vi "CLD 9 Step Sequencer Express Timer Solution.vi"() -> ()   [LabVIEW 2019]
doc: "CLD 9\n\nThis solution uses the Express VI Elapsed Time as a method for timing the changing of states. All of the stat data is hard coded for this exercise."
uses:
  CLD 9 Timer Enum.ctl
panel:
  out "Current Step Time":dbl
  out "Elapsed Time (s)":dbl format="%#.1g"
  out "Step 3":bool
  out "Step 2":bool
  out "Step 1":bool
  out "Time Has Elapsed":bool
  in  "Auto Reset":bool=TRUE
  in  "Reset Button":bool
  in  "Stop VI":bool
  out "error out":errorcluster
  in  "error in":errorcluster
  in  "Time Target (s)":dbl
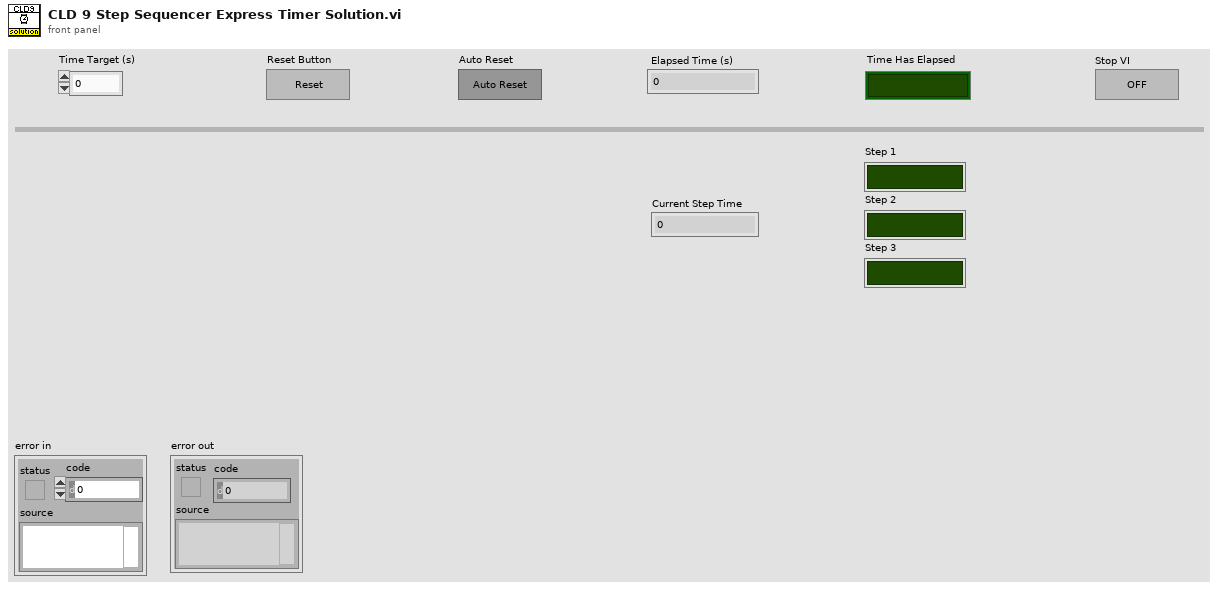
[diagram p1: front panel]
types:
  T1 = typedef "CLD 9 Timer Enum.ctl" = enum16{"Start Step One", "Run Step One", "Start Step Two", "Run Step Two", "Start Step Three", "Run Step Three"}
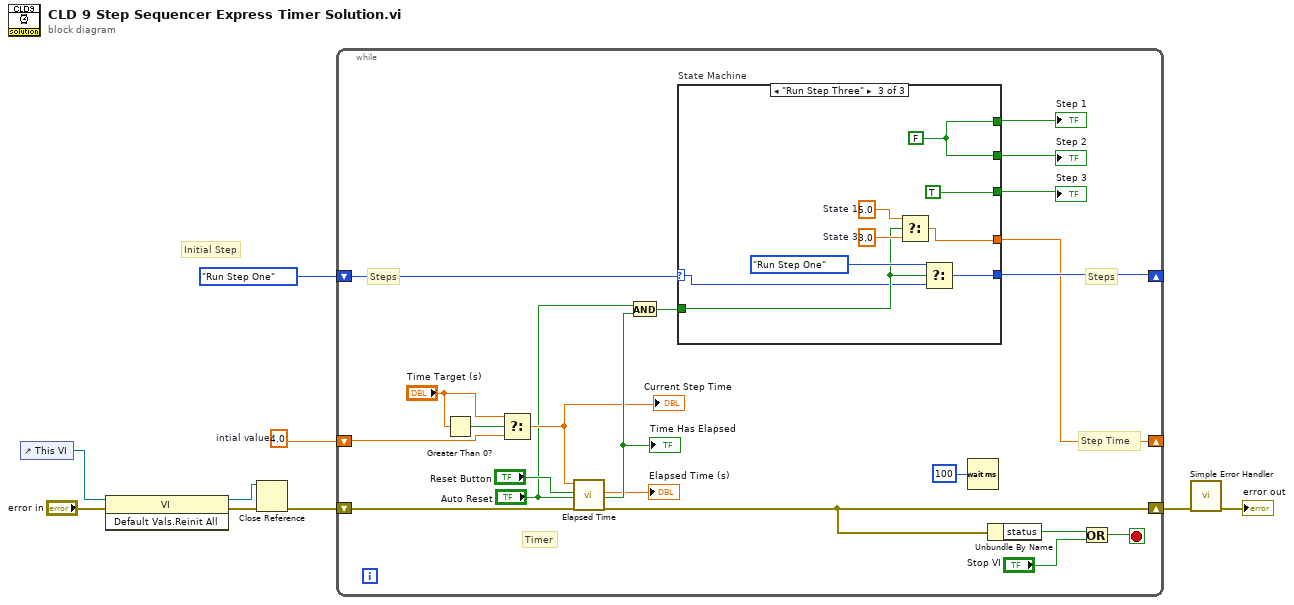
[diagram p0: block diagram]
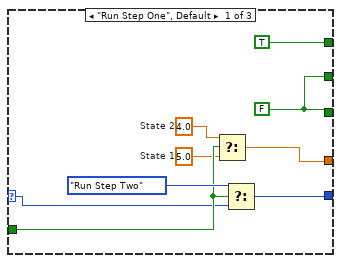
[diagram p2: hidden frame]
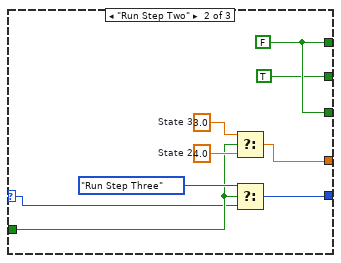
[diagram p3: hidden frame]
diagram:
  w1 = 4.0  # intial value
  # "Initial Step"
  n1 = control-ref of="This VI"() -> (w5:refnum<vi>)
  n2 = invoke class="VI" method="Default Vals.Reinit All"(reference=w5, error in="error in") -> (reference out=w3:refnum<vi>, error out=w6:errorcluster)  [unwired: 1 in, 1 out]
  n3 = Close Reference(reference=w3, error in (no error)=w6) -> (error out=w4:errorcluster)
  n4 = while {
    shift-right: [w13] -> w8
    shift-left: w4 -> [w28]
    shift-right: [w26] -> _
    shift-left: CLD_9_Timer_Enum."Run Step One" ("Enum") -> [w25]
    shift-right: [w17] -> _
    shift-left: w1 -> [w16]
    stop <- w12 stop-if-true
    # "Timer"
    # "Steps"
    # "Steps"
    # "Step Time"
    n5 = Greater Than 0?(x="Time Target (s)") -> (x > 0?=w20:bool)
    n6 = Select(t="Time Target (s)", s=w20, f=w16) -> (s? t:f=w18:dbl)
    "Current Step Time" <- w18
    n7 = call "Elapsed Time"("Time Target (s)"=w18, "Reset"="Reset Button", "Auto Reset"="Auto Reset", "error in (no error)"=w28) -> ("Elapsed Time (s)"=→"Elapsed Time (s)":dbl, "Time has Elapsed"=w24:bool, "error out"=w13:errorcluster)  [unwired: 8 in, 5 out]
    "Time Has Elapsed" <- w24
    n8 = And(x="Auto Reset", y=w24) -> (x .and. y?=w15:bool)
    n9 = case "State Machine" shown="\"Run Step Three\"" w25 {
      selector: w25 -> [w31 w40 w49]
      tunnel: [w36 w47 w56] -> w26
      tunnel: w15 -> [w35 w41 w50]
      tunnel: [TRUE w46 w54] -> w23
      tunnel: [w38 TRUE w54] -> w22
      tunnel: [w38 w46 TRUE] -> w21
      tunnel: [w32 w42 w51] -> w17
      frame "Run Step One", Default {
        w33 = 5.0  # State 1
        w34 = 4.0  # State 2
        w38 = FALSE
        n10 = Select(t=w34, s=w35, f=w33) -> (s? t:f=w32:dbl)
        n11 = Select(t=CLD_9_Timer_Enum."Run Step Two", s=w35, f=w31) -> (s? t:f=w36:T1)
      }
      frame "Run Step Two" {
        w43 = 4.0  # State 2
        w44 = 3.0  # State 3
        w46 = FALSE
        n12 = Select(t=w44, s=w41, f=w43) -> (s? t:f=w42:dbl)
        n13 = Select(t=CLD_9_Timer_Enum."Run Step Three", s=w41, f=w40) -> (s? t:f=w47:T1)
      }
      frame "Run Step Three" {
        w52 = 3.0  # State 3
        w53 = 5.0  # State 1
        w54 = FALSE
        n14 = Select(t=w53, s=w50, f=w52) -> (s? t:f=w51:dbl)
        n15 = Select(t=CLD_9_Timer_Enum."Run Step One", s=w50, f=w49) -> (s? t:f=w56:T1)
      }
    }
    "Step 1" <- w23
    "Step 2" <- w22
    "Step 3" <- w21
    n16 = Wait (ms)(milliseconds to wait=u32 100) -> ()  [unwired: 1 out]
    n17 = Unbundle By Name(w13) -> ("status"=w11:bool)
    n18 = Or(x=w11, y="Stop VI") -> (x .or. y?=w12:bool)
  }
  n19 = call <vilib>:"Simple Error Handler.vi"("error in (no error)"=w8) -> ("error out"=→"error out":errorcluster)  [unwired: 4 in, 4 out]
